vi "Count Up U16.vi"(0 "increment":bool=TRUE, 1 "reset":bool) -> (4 "count out":u16)   [LabVIEW 2015, in "Engine Simulation Toolkit.lvlib"]
uses:
  Engine Simulation Toolkit.lvlib
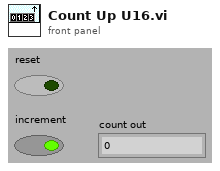
[diagram p1: front panel]
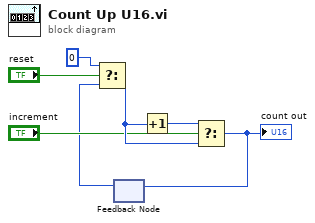
[diagram p0: block diagram]
diagram:
  n1 = feedback #1() -> (w2:u16)  [unwired: 1 in]
  n2 = Select(t=u16 0 ("count in"), s="reset", f=w2) -> (s? t:f=w6:u16)
  n3 = Increment(x=w6) -> (x+1=w7:u16)
  n4 = Select(t=w7, s="increment", f=w6) -> (s? t:f=w1:u16)
  "count out" <- w1
  n5 = feedback-in #1(w1) -> ()
